vi "base_node.vi"() -> ()   [LabVIEW 2018]
panel:
  in  "I am:":enum32{"Training", "Testing", "Implementing"}(radio)
  # "Neural Network Base Node"
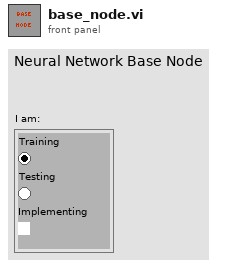
[diagram p1: front panel]
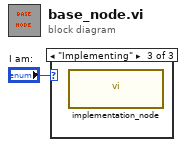
[diagram p0: block diagram]
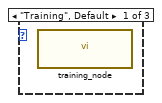
[diagram p2: hidden frame]
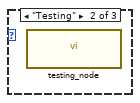
[diagram p3: hidden frame]
diagram:
  n1 = case shown="\"Implementing\"" "I am:" {
    frame "Training", Default {
      n2 = call "training_node.vi"() -> ()  [unwired: 12 in]
    }
    frame "Testing" {
      n3 = call "testing_node.vi"() -> ()  [unwired: 12 in]
    }
    frame "Implementing" {
      n4 = call "implementation_node.vi"() -> ()  [unwired: 12 in]
    }
  }
